vi "Create.vi"(8 "error in":errorcluster, 9 "Header Footer OffsetCluster":T2={"Header Offset"=100.0, "Footer Offset"=300.0, "Margin"={"Left"=40.0, "Right"=40.0, "Top"=100.0, "Bottom"=300.0}}, 10 "PDF Details":T3={"Title"="Advanced Header/Footer", "Subject"="", "Keywords"="", "Author"="Simplicity AI", "Creator"="Simplicity AI PDF API"}, 11 "Context In":refnum<class "Context.lvclass">) -> (0 "error out":errorcluster, 3 "Context Out":refnum<class "Context.lvclass">)   [LabVIEW 2020, in "PDF Interface.lvlib" / "PDF Interface Helper.lvlib"]
doc: "Creates the PDF document basic layout and opens a new PDF file on disk."
uses:
  <vilib>/Simplicity AI/SAI_PDF_API/Classes/Context/Context.lvclass
  <vilib>/Simplicity AI/SAI_PDF_API/Classes/Context/Controls/SAI_PDF_PDF Details.ctl
  <vilib>/Simplicity AI/SAI_PDF_API/Classes/Context/Controls/SAI_PDF_Margins.ctl
  PDF Interface Helper.lvlib
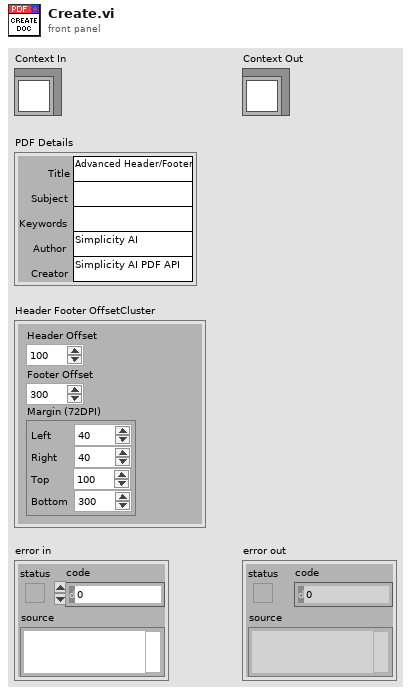
[diagram p1: front panel]
types:
  T1 = typedef "SAI_PDF_Toolkit.lvlib/Context.lvclass/SAI_PDF_Margins.ctl" = cluster{"Left":sgl, "Right":sgl, "Top":sgl, "Bottom":sgl}
  T2 = cluster{"Header Offset":sgl, "Footer Offset":sgl, "Margin":T1}
  T3 = typedef "SAI_PDF_Toolkit.lvlib/Context.lvclass/SAI_PDF_PDF Details.ctl" = cluster{"Title":string, "Subject":string, "Keywords":string, "Author":string, "Creator":string}
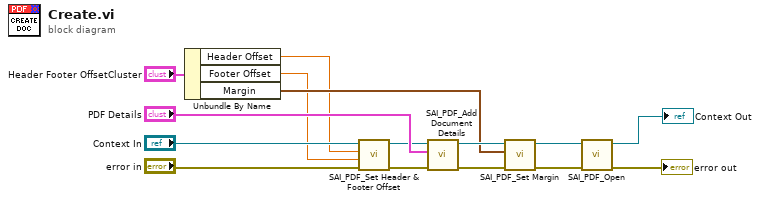
[diagram p0: block diagram]
diagram:
  n1 = Unbundle By Name("Header Footer OffsetCluster") -> ("Header Offset"=w2:sgl, "Footer Offset"=w1:sgl, "Margin"=w3:T1)
  n2 = call <vilib>:"SAI_PDF_Set Header & Footer Offset.vi"("error in"="error in", "Footer Offset"=w1, "Header Offset"=w2, "Context In"="Context In") -> ("error out"=w12:errorcluster, "Context Out"=w14:refnum<class "Context.lvclass">)  [unwired: 6 out]
  n3 = call <vilib>:"SAI_PDF_Add Document Details.vi"("error in"=w12, "PDF Details"="PDF Details", "Context In"=w14) -> ("error out"=w8:errorcluster, "Context Out"=w9:refnum<class "Context.lvclass">)  [unwired: 7 out]
  n4 = call <vilib>:"SAI_PDF_Set Margin.vi"("error in"=w8, "Margin"=w3, "Context In"=w9) -> ("error out"=w10:errorcluster, "Context Out"=w11:refnum<class "Context.lvclass">)  [unwired: 7 out]
  n5 = call <vilib>:"SAI_PDF_Open.vi"("error in"=w10, "Context In"=w11) -> ("error out"=→"error out":errorcluster, "Context Out"=→"Context Out":refnum<class "Context.lvclass">)  [unwired: 3 in, 5 out]
